vi "Luhn_CS_Check.vi"(5 "string":string) -> (0 "error out":errorcluster, 2 "Passed":bool)   [LabVIEW 2012]
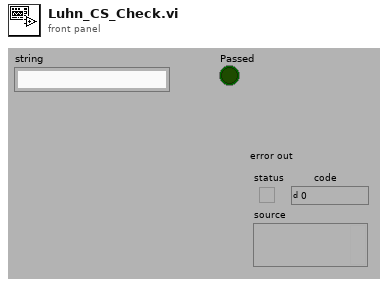
[diagram p1: front panel]
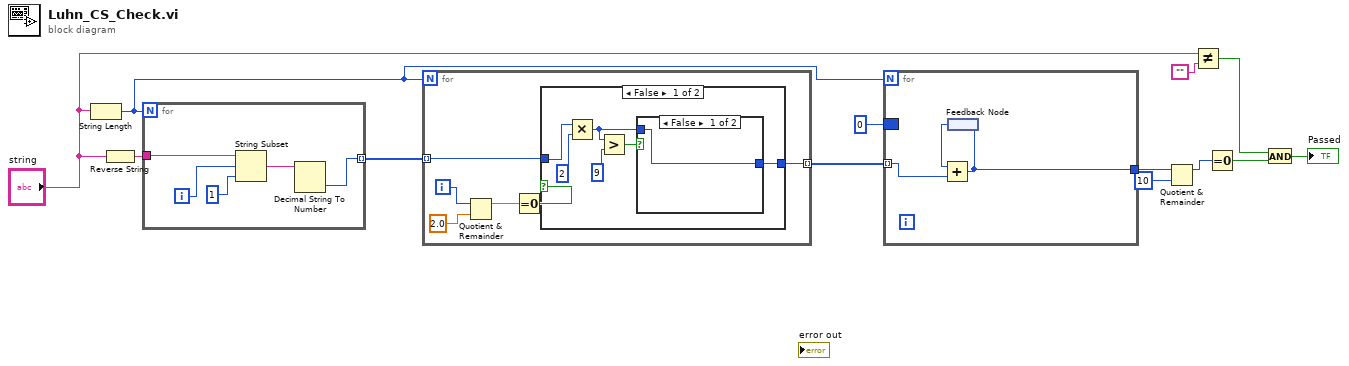
[diagram p0: block diagram]
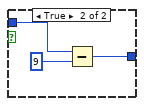
[diagram p2: hidden frame]
diagram:
  n1 = String Length(string="string") -> (length=w10:i32)
  n2 = Reverse String(1:"string") -> (0:w13:string)
  n3 = for {
    N: w10 -> [_]
    tunnel: w13 -> [w14]
    tunnel: [w15] -> w12 mode=indexing
    i -> [w16]
    n4 = String Subset(string=w14, offset (0)=w16, length (rest)=1 ("length (rest)")) -> (substring=w17:string)
    n5 = Decimal String To Number(string=w17) -> (number=w15:i32)  [unwired: 2 in, 1 out]
  }
  n6 = for {
    N: w10 -> [_]
    tunnel: w12 -> [w20] mode=indexing
    tunnel: [w19] -> w11 mode=indexing
    i -> [w23]
    n7 = Quotient & Remainder(x=w23, y=2.0) -> (x-y*floor(x/y)=w22:dbl)  [unwired: 1 out]
    n8 = Equal To 0?(x=w22) -> (x = 0?=w21:bool)
    n9 = case shown="False" w21 {
      tunnel: w20 -> [w30 w35]
      tunnel: [w25 w35] -> w19
      frame False {
        n10 = Multiply(x=w30, y=2) -> (x*y=w26:i32)
        n11 = Greater?(x=w26, y=9) -> (0:w27:bool)
        n12 = case shown="False" w27 {
          tunnel: w26 -> [w31 w34]
          tunnel: [w31 w32] -> w25
          frame False {
          }
          frame True {
            n13 = Subtract(x=w34, y=9) -> (x-y=w32:i32)
          }
        }
      }
      frame True {
      }
    }
  }
  n14 = for {
    N: w10 -> [_]
    tunnel: w11 -> [w37] mode=indexing
    tunnel: [w36] -> w8
    border: 0 -> [_]
    n15 = feedback #1() -> (w38:i32)
    n16 = Add(x=w38, y=w37) -> (x+y=w36:i32)
    n17 = feedback-in #1(w36) -> ()
  }
  n18 = Quotient & Remainder(x=w8, y=10) -> (x-y*floor(x/y)=w6:i32)  [unwired: 1 out]
  n19 = Not Equal?(x="string", y="") -> (x != y?=w1:bool)
  n20 = Equal To 0?(x=w6) -> (x = 0?=w5:bool)
  n21 = And(x=w1, y=w5) -> (x .and. y?=→"Passed":bool)
